vi "3. Panel Events.vi"() -> ()   [LabVIEW 2020, in "1. Basic Panels.lvlib"]
doc: "Panel Events Example.\n----\nCopyright: MGI 2017\nAuthor: Derek Trepanier"
uses:
  1. Basic Panels.lvlib
  <vilib>/MGI/Panel Manager/Panel/Window Position/Reference Position/Offset/Absolute Offset/Absolute Offset.lvclass/Absolute Offset.ctl
  <vilib>/MGI/Panel Manager/Panel/Window Position/Reference Position/Offset/Absolute Offset/Absolute Offset.vi
  <vilib>/MGI/Panel Manager/Panel/Panel/Subpanel/Subpanel.lvclass
  C:/Program Files/National Instruments/LabVIEW 2020/vi.lib/MGI/Panel Manager/Panel/Panel/Panel.lvclass
  <vilib>/MGI/Panel Manager/Panel/Panel/Window/Window.lvclass
  <vilib>/MGI/Panel Manager/Panel/Window Position/Reference Position/Offset/Absolute Offset/Absolute Offset.lvclass
  C:/Program Files/National Instruments/LabVIEW 2020/vi.lib/MGI/Panel Manager/Panel/Window Position/Reference Position/Offset/Offset.lvclass
  <vilib>/MGI/Panel Manager/Panel/Window Position/Reference Position/Ref Display/Ref Display.lvclass
  C:/Program Files/National Instruments/LabVIEW 2020/vi.lib/MGI/Panel Manager/Panel/Window Position/Window Position.lvclass
  <vilib>/MGI/Panel Manager/Panel/Panel/Subpanel/Subpanel.vi
  <vilib>/MGI/Panel Manager/Panel/Window Position/Reference Position/Ref Display/Ref Display.vi
  <vilib>/MGI/Panel Manager/Panel/Panel/Window/Window.vi
  <vilib>/MGI/Panel Manager/Panel/Panel.lvlib
  C:/Program Files/National Instruments/LabVIEW 2020/vi.lib/MGI/Panel Manager/Panel/Window Position/Reference Position/Offset/Absolute Offset/Absolute Offset.lvclass
  C:/Program Files/National Instruments/LabVIEW 2020/vi.lib/MGI/Panel Manager/Panel/Window Position/Reference Position/Reference Position.lvclass
  C:/Program Files/National Instruments/LabVIEW 2020/vi.lib/MGI/Panel Manager/Panel/Window Position/Reference Position/Ref Display/Ref Display.lvclass
panel:
  in  "All Panels":i32(listbox)
  in  "New Subpanel":bool
  in  "New Window":bool
  # "No Panels are Active"
  # "Run this VI to view the Panel Events Demo"
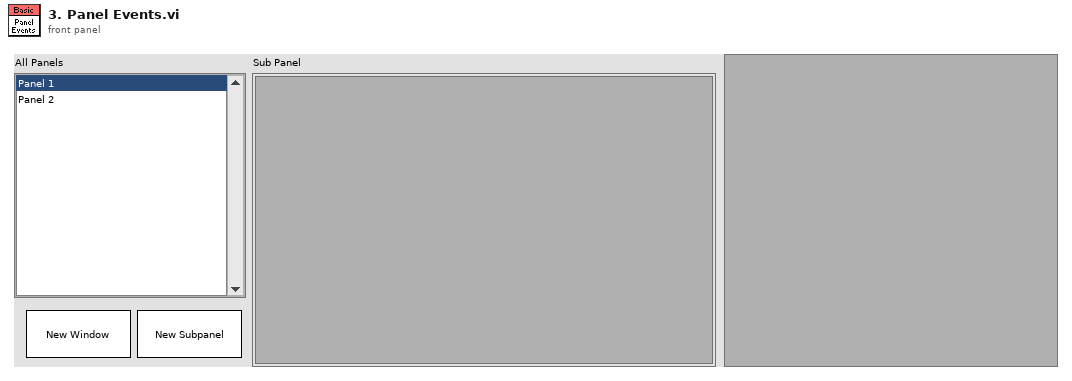
[diagram p1: front panel]
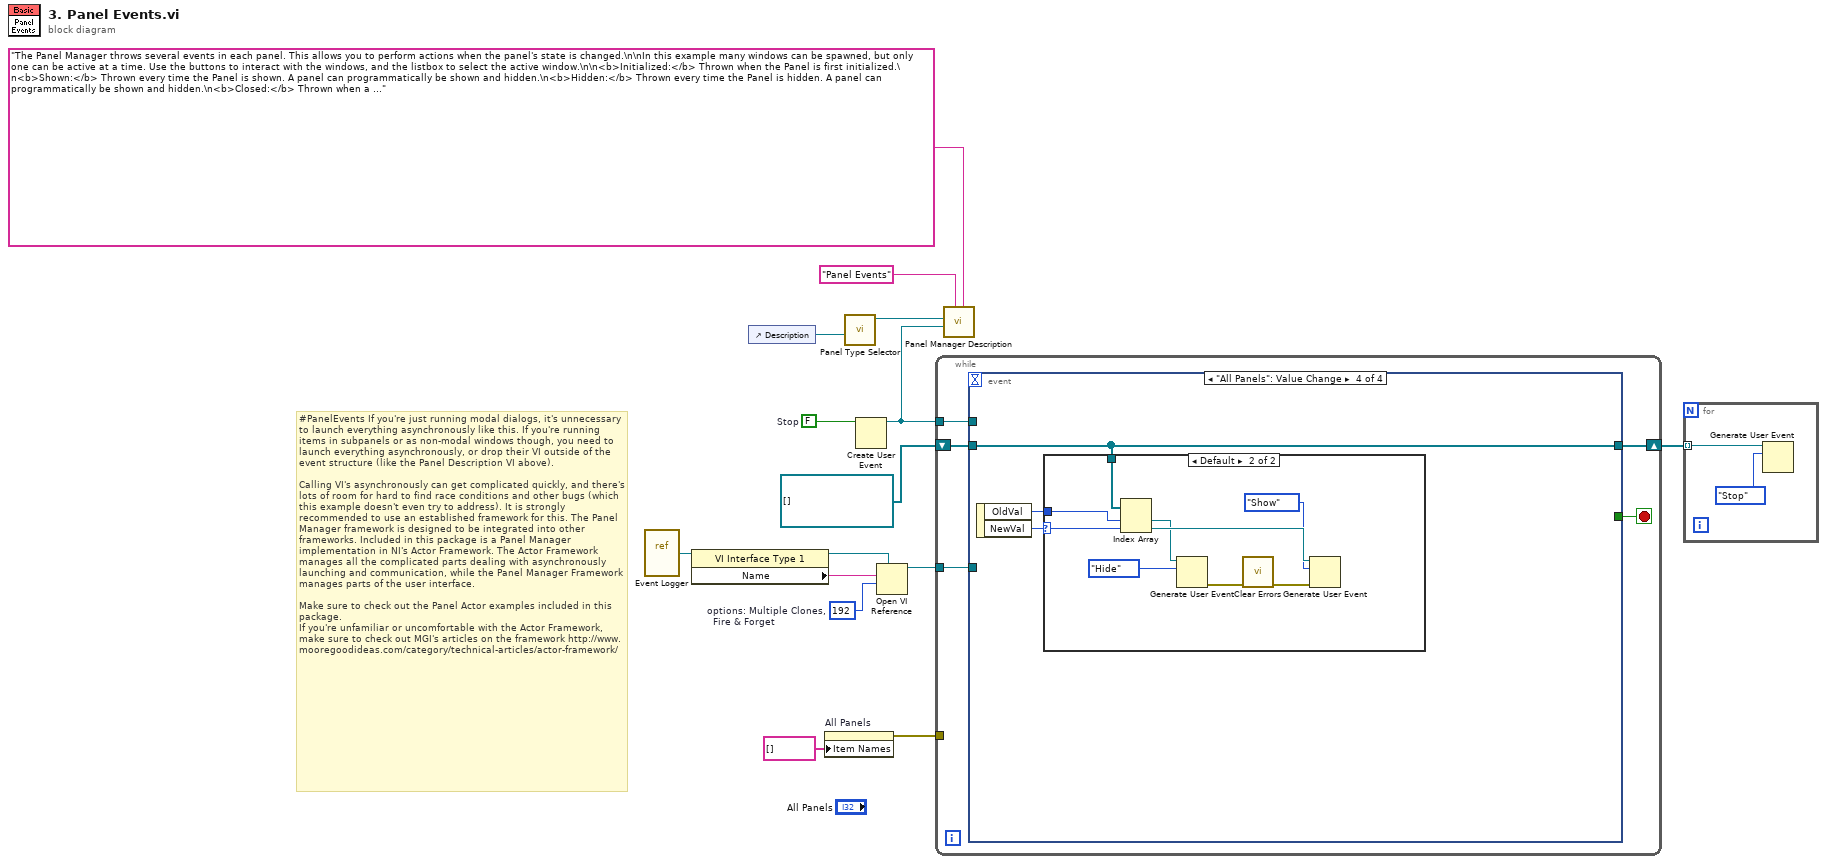
[diagram p0: block diagram]
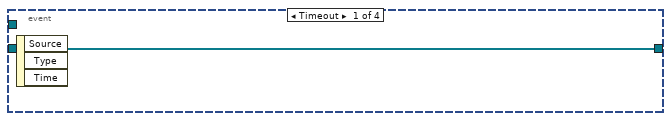
[diagram p2: hidden frame]
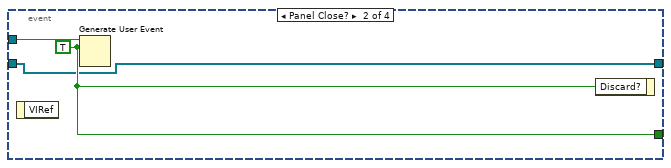
[diagram p3: hidden frame]
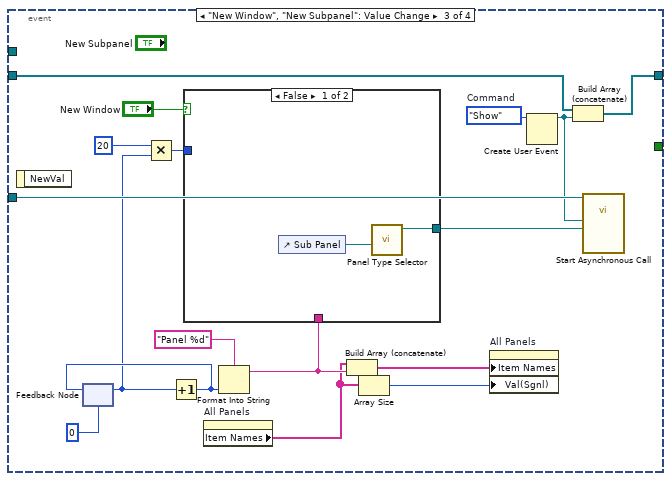
[diagram p4: hidden frame]
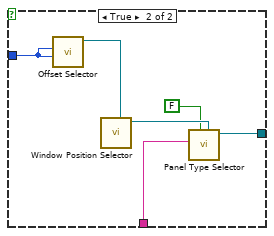
[diagram p5: hidden frame]
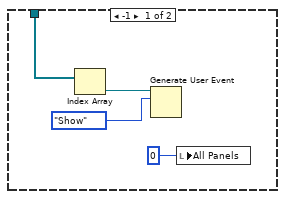
[diagram p6: hidden frame]
diagram:
  w4 = refnum<user-event>[] [] items=["Show", "Hide", "Stop"]
  w6 = 192  # options: Multiple Clones,   Fire & Forget
  w14 = FALSE  # Stop
  # "#PanelEvents If you're just running modal dialogs, it's unnecessary to launch everything asynchronously like this. If you're running items in subpanels or as non-modal windows though, you need to launch everything asynchronously, or drop their VI outside of the event structure (like the Panel Description VI above).\n\nCalling VI's asynchronously can get complicated quickly, and there's lots of room for hard to find race conditions and other bugs (which this example doesn't even try to address). It is strongly recommended to use an established framework for this. The Panel Manager framework is designed to be integrated into other frameworks. Included in this package is a Panel Manager implementation in NI's Actor Framework. The Actor Framework manages all the complicated parts dealing with asynchronously launching and communication, while the Panel Manager Framework manages parts of the user interface.\n\nMake sure to check out the Panel Actor examples included in this package.\nIf you're unfamiliar or uncomfortable with the Actor Framework, make sure to check out MGI's articles on the framework http://www.mooregoodideas.com/category/technical-articles/actor-framework/"
  n1 = vi-ref "Event Logger.vi"() -> (w9:refnum<vi>)
  n2 = property class="VI Interface Type 1"(reference=w9) -> (reference out=w8:refnum<vi>, "Name"=w7:string)  [unwired: 1 in, 1 out]
  n3 = control-ref of="Description"() -> (w12:refnum<vi>)
  n4 = property on="All Panels" class="LstBox (strict)"("Item Names"=string[] []) -> (error out=w2:errorcluster)  [unwired: 2 in, 1 out]
  n5 = call-poly <vilib>:"Panel Type Selector.vi"("Sub Panel"=w12) -> ("Subpanel Out"=w15:refnum<class "Subpanel.lvclass">)  [unwired: 9 in, 1 out]
  n6 = Create User Event(user event datatype=w14) -> (user event=w11:refnum<user-event>)  [unwired: 1 in, 1 out]
  n7 = Open VI Reference(type specifier VI Refnum (for type only)=w8, vi path=w7, options=w6) -> (vi reference=w5:refnum<vi>)  [unwired: 3 in, 1 out]
  n8 = while {
    tunnel: w11 -> [w20]
    tunnel: w5 -> [w18]
    shift-right: [w17] -> w3
    shift-left: w4 -> [w16]
    tunnel: w2 -> [_]
    stop <- w19 stop-if-true
    n9 = event shown="[3] \"All Panels\": Value Change" {
      selector: _ -> [_ _ _ _]
      dyn-events: _ -> [_ _ _ _]
      timeout: _ -> [_ _ _ _]
      tunnel: w20 -> [_ w24 _ _]
      tunnel: [_ w23 _ _] -> w19
      tunnel: w18 -> [_ _ w41 _]
      tunnel: [w21 w22 w35 w52] -> w17
      tunnel: w16 -> [w21 w22 w34 w52]
      event Timeout {
        n10 = event-data() -> ()  [unwired: 1 in, 3 out]
      }
      event Panel Close? {
        w23 = TRUE ("event data")
        n11 = event-data() -> ()  [unwired: 1 in, 1 out]
        n12 = Generate User Event(user event=w24, event data cluster=w23) -> ()  [unwired: 2 in, 2 out]
        n13 = event-data("Discard?"=w23) -> ()  [unwired: 1 in, 1 out]
      }
      event "New Window", "New Subpanel": Value Change {
        w37 = enum16{"Show", "Hide", "Stop"}."Show"  # Command
        n14 = event-data() -> ()  [unwired: 1 in, 1 out]
        n15 = feedback #1(0) -> (w27:i32)
        n16 = Multiply(x=20, y=w27) -> (x*y=w28:i32)
        n17 = Increment(x=w27) -> (x+1=w29:i32)
        n18 = feedback-in #1(w29) -> ()
        n19 = property on="All Panels" class="LstBox (strict)"() -> ("Item Names"=w31:string[])  [unwired: 2 in, 2 out]
        n20 = Format Into String(format string="Panel %d", w29) -> (resulting string=w33:string)  [unwired: 2 in, 1 out]
        n21 = case shown="False" "New Window" {
          tunnel: [w43 w49] -> w40
          tunnel: w33 -> [_ w48]
          tunnel: w28 -> [_ w44]
          frame False {
            n22 = control-ref of="Sub Panel"() -> (w42:refnum<vi>)
            n23 = call-poly <vilib>:"Panel Type Selector.vi"("Sub Panel"=w42) -> ("Subpanel Out"=w43:refnum<class "Subpanel.lvclass">)  [unwired: 9 in, 1 out]
          }
          frame True {
            n24 = call-poly <vilib>:"Offset Selector.vi"("Vertical"=w44, "Horizontal"=w44) -> ("Absolute Offset Out"=w45:refnum<class "Absolute Offset.lvclass">)  [unwired: 8 in, 1 out]
            n25 = call-poly <vilib>:"Window Position Selector.vi"("Offset"=w45) -> ("Ref Display out"=w47:refnum<class "Ref Display.lvclass">)  [unwired: 9 in, 1 out]
            n26 = call-poly <vilib>:"Panel Type Selector.vi"("Window Position"=w47, "Autoshow? (T)"=FALSE, "Default Title"=w48) -> ("Window out"=w49:refnum<class "Window.lvclass">)  [unwired: 7 in, 1 out]
          }
        }
        n27 = Build Array (concatenate)(w31, w33) -> (w32:string[])
        n28 = Array Size(array=w31) -> (size(s)=w30:i32)
        n29 = property on="All Panels" class="LstBox (strict)"("Item Names"=w32, "Val(Sgnl)"=w30) -> ()  [unwired: 2 in, 2 out]
        n30 = Create User Event(user event datatype=w37) -> (user event=w36:refnum<user-event>)  [unwired: 1 in, 1 out]
        n31 = Build Array (concatenate)(w34, w36) -> (w35:refnum<user-event>[])
        n32 = call-by-ref "Start Asynchronous Call"(reference=w41, "Panel"=w40, "user event out"=w36) -> ()  [unwired: 11 in, 2 out]
      }
      event "All Panels": Value Change {
        n33 = event-data() -> ("OldVal"=w51:i32, "NewVal"=w50:i32)  [unwired: 1 in]
        n34 = case shown="Default" w50 {
          selector: w50 -> [_ w64]
          tunnel: w52 -> [w56 w65]
          tunnel: w51 -> [_ w61]
          frame -1 {
            n35 = Index Array(array=w56) -> (element=w54:refnum<user-event>)  [unwired: 1 in]
            n36 = Generate User Event(user event=w54, event data cluster=enum16{"Show", "Hide", "Stop"}."Show" ("event data")) -> ()  [unwired: 2 in, 2 out]
            n37 = local write "All Panels"(0 ("All Windows")) -> ()
          }
          frame Default {
            n38 = Index Array(array=w65, index #1=w61, index #2=w64) -> (element #1=w60:refnum<user-event>, element #2=w63:refnum<user-event>)
            n39 = Generate User Event(user event=w60, event data cluster=enum16{"Show", "Hide", "Stop"}."Hide" ("event data")) -> (error out=w59:errorcluster)  [unwired: 2 in, 1 out]
            n40 = call <vilib>:"Clear Errors.vi"("error in (no error)"=w59) -> ("error out"=w58:errorcluster)  [unwired: 5 in, 1 out]
            n41 = Generate User Event(user event=w63, event data cluster=enum16{"Show", "Hide", "Stop"}."Show" ("event data"), error in=w58) -> ()  [unwired: 1 in, 2 out]
          }
        }
      }
    }
  }
  n42 = call "Panel Manager Description.vi"("Description"="The Panel Manager throws several events in each panel. This allows you to perform actions when the panel's state is changed.\n\nIn this example many windows can be spawned, but only one can be active at a time. Use the buttons to interact with the windows, and the listbox to select the active window.\n\n<b>Initialized:</b> Thrown when the Panel is first initialized.\n<b>Shown:</b> Thrown every time the Panel is shown. A panel can programmatically be shown and hidden.\n<b>Hidden:</b> Thrown every time the Panel is hidden. A panel can programmatically be shown and hidden.\n<b>Closed:</b> Thrown when a Panel Object is closed.\n\n<b>Note:</b> Panel Events are extremly useful when working with Panel Actors. See the \"Panel Actor: Changing Panel Types\" example for more demonstrations of panel events.\n\nSee the #PanelEvents bookmark for more info." ("Description Title"), "Description Title"="Panel Events", "Stop Event"=w11, "Panel"=w15) -> ()  [unwired: 7 in, 1 out]
  n43 = for {
    tunnel: w3 -> [w67] mode=indexing
    n44 = Generate User Event(user event=w67, event data cluster=enum16{"Show", "Hide", "Stop"}."Stop" ("event data")) -> ()  [unwired: 2 in, 2 out]
  }
